vi "Summator.vi"(6 "Store":T1=enum."sum_up", 8 "error in (no error)":errorcluster, 10 "Waveform in":waveform(dbl), 11 "RFID system in":refnum<class "RFID system.lvclass">) -> (0 "error out":errorcluster, 2 "Waveform out":waveform(dbl), 3 "RFID system out":refnum<class "RFID system.lvclass">)   [LabVIEW 2019, in "RFID system.lvclass"]
uses:
  RFID system.lvclass
  TypeDef/Store.ctl
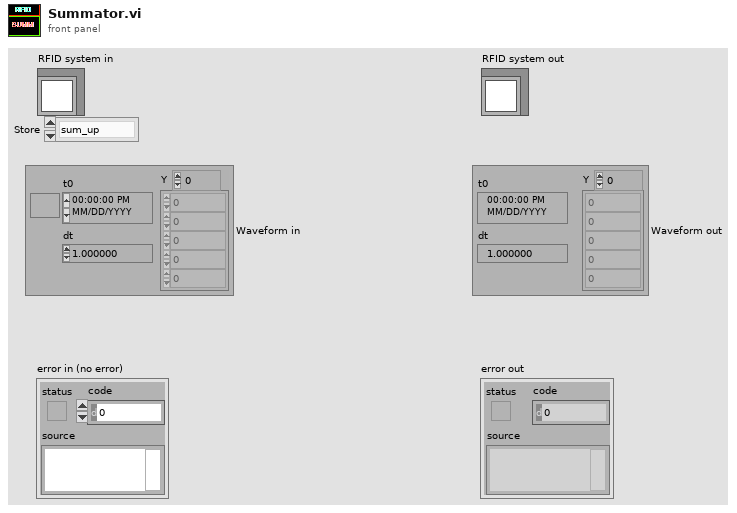
[diagram p1: front panel]
types:
  T1 = typedef "Store.ctl" = enum16{"envelope", "noise", "demSubCar", "CH_frame", "Decode", "demodulate", "in", "out", "sum", "subCarrier", "frame", "command", "encode", "modulate", "encode_UP", "modulate_up", "demod_up", "envelop_up", "sum_up", "out_up", "in_up"}
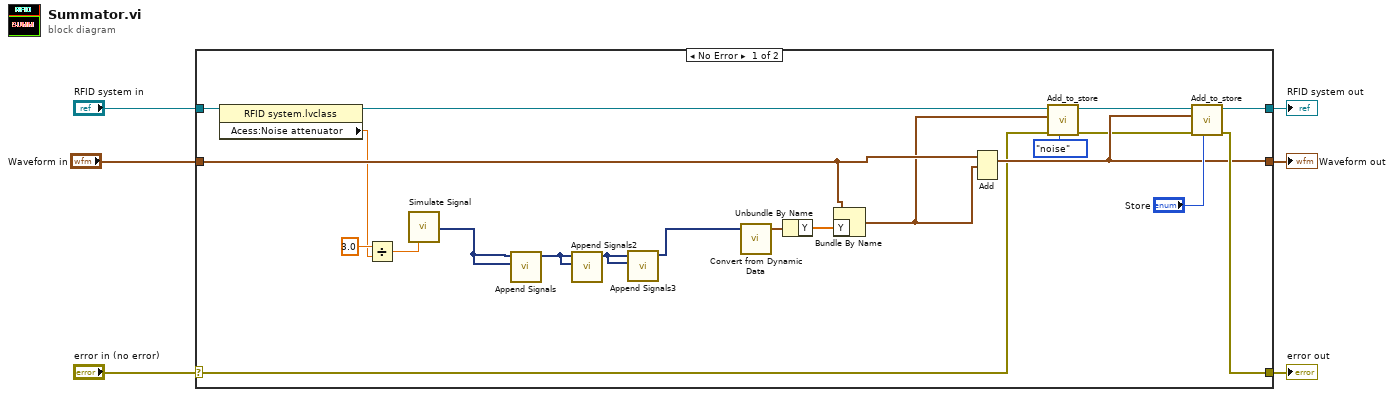
[diagram p0: block diagram]
diagram:
  n1 = case shown="No Error" "error in (no error)" {
    selector: "error in (no error)" -> [w16 w29]
    tunnel: [w23 w29] -> w5
    tunnel: [w24 w30] -> w3
    tunnel: "RFID system in" -> [w19 w30]
    tunnel: "Waveform in" -> [w20 w28]
    tunnel: [w21 w28] -> w1
    frame No Error {
      n2 = property class="RFID system.lvclass"(reference=w19) -> (reference out=w11:refnum<class "RFID system.lvclass">, "Acess:Noise attenuator"=w7:dbl)  [unwired: 1 in, 1 out]
      n3 = Divide(x=3.0 ("y"), y=w7) -> (x/y=w9:dbl)
      n4 = call "Simulate Signal"("Standard deviation"=w9) -> ("Sine with Gaussian Noise"=w25:dynamicdata)  [unwired: 13 in, 1 out]
      n5 = call "Append Signals"("Input Signal B"=w25, "Input Signal A"=w25) -> ("Appended Signals"=w13:dynamicdata)  [unwired: 8 in, 1 out]
      n6 = call "Append Signals2"("Input Signal B"=w13, "Input Signal A"=w13) -> ("Appended Signals"=w12:dynamicdata)  [unwired: 8 in, 1 out]
      n7 = call "Append Signals3"("Input Signal B"=w12, "Input Signal A"=w12) -> ("Appended Signals"=w10:dynamicdata)  [unwired: 8 in, 1 out]
      n8 = call "Convert from Dynamic Data"("Dynamic Data Type"=w10) -> ("Waveform"=w27:waveform(dbl))  [unwired: 3 in]
      n9 = Unbundle By Name(w27) -> ("Y"=w26:dbl[])
      n10 = Bundle By Name(cluster=w20, "Y"=w26) -> (w17:waveform(dbl))
      n11 = Add(1:w17, 2:w20) -> (0:w21:waveform(dbl))  [unwired: 1 in, 1 out]
      n12 = call "Add_to_store.vi"("Store"=Store."noise", "error in (no error)"=w16, "Waveform"=w17, "RFID system in"=w11) -> ("error out"=w15:errorcluster, "RFID system out"=w18:refnum<class "RFID system.lvclass">)  [unwired: 6 in]
      n13 = call "Add_to_store.vi"("Store"="Store", "error in (no error)"=w15, "Waveform"=w21, "RFID system in"=w18) -> ("error out"=w23:errorcluster, "RFID system out"=w24:refnum<class "RFID system.lvclass">)  [unwired: 6 in]
    }
    frame Error {
      # "Wire the error cluster across even in the \"No Error\"\ncase so that warnings get propagated."
    }
  }
  "error out" <- w5
  "RFID system out" <- w3
  "Waveform out" <- w1
